vi "_Write to Pipe BG.vi"(9 "fd":u64, 10 "path":path, 11 "Password":string) -> ()   [LabVIEW 2020, in "NI_SSH.lvlib" / "OpenSSH Client.lvclass"]
uses:
  <vilib>/net/SSH/Client/OpenSSH/OpenSSH Client.lvclass
  lviosrg.dll
  <vilib>/Subprocess/Subprocess/Subprocess.lvclass
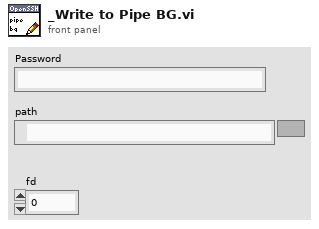
[diagram p1: front panel]
types:
  T1 = enum16{"open", "replace", "create", "open or create", "replace or create", "replace or create with confirmation"}
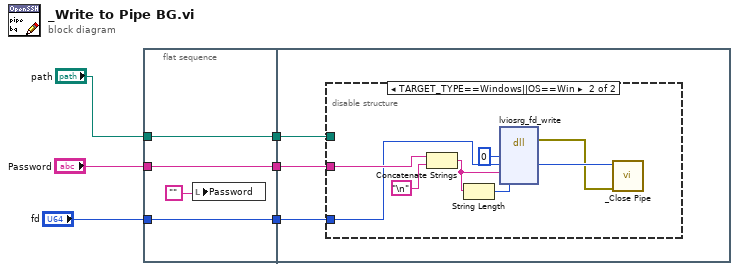
[diagram p0: block diagram]
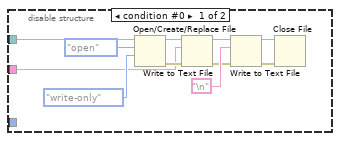
[diagram p2: hidden frame]
diagram:
  n1 = flat-sequence {
    tunnel: "Password" -> [w9]
    tunnel: "path" -> [w10]
    tunnel: [w10] -> w4
    tunnel: [w9] -> w3
    tunnel: [w7] -> w2
    tunnel: "fd" -> [w7]
    tunnel: w4 -> [w13]
    tunnel: w3 -> [w12]
    tunnel: w2 -> [w11]
    frame #0 {
      n2 = local write "Password"("") -> ()
    }
    frame #1 {
      n3 = disable-structure shown="TARGET_TYPE==Windows||OS==Win" {
        disable-tunnel: w13 -> [w21 _]
        disable-tunnel: w12 -> [w14 w32]
        disable-tunnel: w11 -> [_ w30]
        frame condition #0 {
          n4 = Open/Create/Replace File(file path (use dialog)=w21, operation (0:open)=T1."open", access (0:read/write)=enum16{"read/write", "read-only", "write-only"}."write-only") -> (refnum out=w22:refnum<file>, error out=w20:errorcluster)  [unwired: 3 in, 1 out]
          n5 = Write to Text File(file (use dialog)=w22, text=w14, error in=w20) -> (refnum out=w15:refnum<file>, error out=w16:errorcluster)  [unwired: 1 in, 1 out]
          n6 = Write to Text File(file (use dialog)=w15, text="\n", error in=w16) -> (refnum out=w17:refnum<file>, error out=w18:errorcluster)  [unwired: 1 in, 1 out]
          n7 = Close File(refnum=w17, error in=w18) -> ()  [unwired: 2 out]
        }
        frame condition #1 (active) {
          n8 = Concatenate Strings(w32, "\n") -> (w28:string)
          n9 = String Length(string=w28) -> (length=w27:i32)
          n10 = dll-call lib="lviosrg.*" fn="lviosrg_fd_write"("errno"=0, "write_fd"=w30, "buf"=w28, "buflen"=w27) -> (error out=w25:errorcluster, "write_fd"=w26:u64)  [unwired: 7 in, 1 out]
          n11 = call <vilib>:"_Close Pipe.vi"("error in"=w25, "fd"=w26) -> ()  [unwired: 8 in, 2 out]
        }
      }
    }
  }
